vi "Failure Info_DL.vi"(8 "error in (no error)":errorcluster, 10 "Failure Info":T2, 11 "DataLogger in":refnum<class "DataLogger.lvclass">) -> (0 "error out":errorcluster, 3 "DataLogger out":refnum<class "DataLogger.lvclass">)   [LabVIEW 2019, in "DataLogger.lvclass"]
uses:
  DataLogger.lvclass
  <vilib>/vision/Image Controls.llb/IMAQ Image.ctl
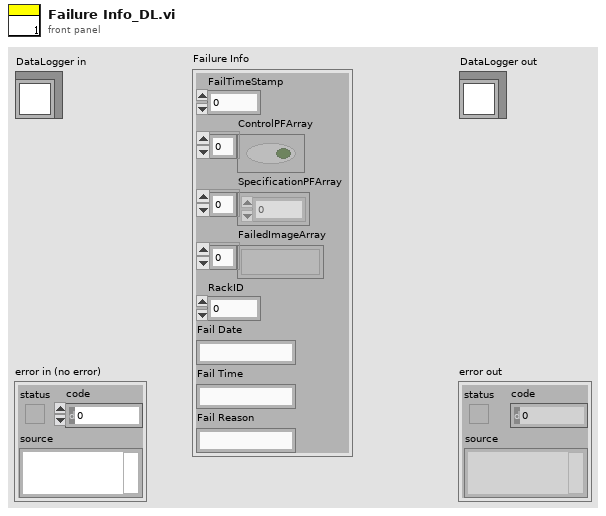
[diagram p1: front panel]
types:
  T1 = typedef "IMAQ Image.ctl" = refnum<image>
  T2 = cluster{"FailTimeStamp":u64, "ControlPFArray":bool[], "SpecificationPFArray":dbl[], "FailedImageArray":T1[], "RackID":u8, "Fail Date":string, "Fail Time":string, "Fail Reason":string}
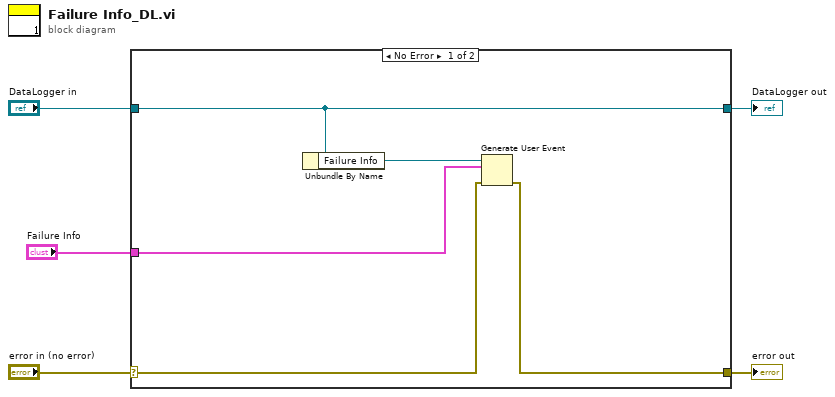
[diagram p0: block diagram]
diagram:
  n1 = case shown="No Error" "error in (no error)" {
    selector: "error in (no error)" -> [w7 w12]
    tunnel: [w6 w12] -> w4
    tunnel: [w10 w11] -> w2
    tunnel: "DataLogger in" -> [w10 w11]
    tunnel: "Failure Info" -> [w8 _]
    frame No Error {
      n2 = Unbundle By Name(w10) -> ("Failure Info"=w9:refnum<user-event>)
      n3 = Generate User Event(user event=w9, event data cluster=w8, error in=w7) -> (error out=w6:errorcluster)  [unwired: 1 in, 1 out]
    }
    frame Error {
    }
  }
  "error out" <- w4
  "DataLogger out" <- w2
